vi "buildconfig.vi"(1 "String":string="home") -> (0 "JSON Tree out (JSON Object)":variant)   [LabVIEW 2017]
uses:
  <vilib>/LVH/i3 JSON/JSON Generation/Create Value Files/Create Value - Object.vi
  <vilib>/LVH/i3 JSON/JSON Generation/Add Object Parameter Files/Add Object Parameter - String.vi
  <vilib>/LVH/i3 JSON/i3-json.lvlib
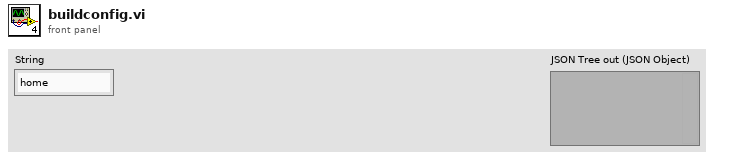
[diagram p1: front panel]
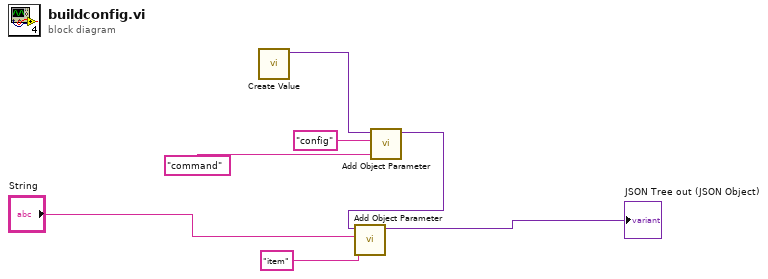
[diagram p0: block diagram]
diagram:
  n1 = call-poly <vilib>:"Create Value.vi"() -> ("JSON Tree"=w7:variant)  [unwired: 10 in, 1 out]
  n2 = call-poly <vilib>:"Add Object Parameter.vi"("Name"="command", "String"="config", "JSON Tree in (JSON Object)"=w7) -> ("JSON Tree out (JSON Object)"=w5:variant)  [unwired: 7 in, 1 out]
  n3 = call-poly <vilib>:"Add Object Parameter.vi"("Name"="item", "String"="String", "JSON Tree in (JSON Object)"=w5) -> ("JSON Tree out (JSON Object)"=→"JSON Tree out (JSON Object)":variant)  [unwired: 7 in, 1 out]
